vi "Set Minimum Pane Size to (0,0).vi"(8 "error in (no error)":errorcluster, 10 "Save VI (T)":bool=TRUE, 11 "vi path":path) -> (0 "error out":errorcluster)   [LabVIEW 2023]
uses:
  <vilib>/Utility/miscctls.llb/LVPointTypeDef.ctl
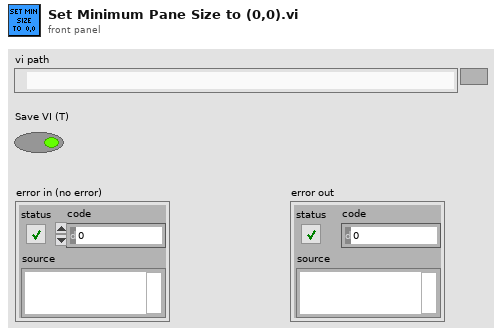
[diagram p1: front panel]
types:
  T1 = typedef "LVPointTypeDef.ctl" = cluster{"Horizontal":i16, "Vertical":i16}
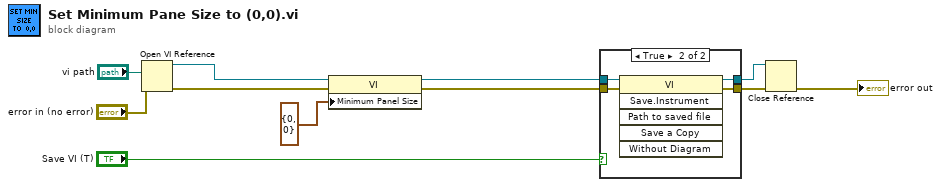
[diagram p0: block diagram]
diagram:
  n1 = Open VI Reference(vi path="vi path", error in (no error)="error in (no error)") -> (vi reference=w6:refnum<vi>, error out=w5:errorcluster)  [unwired: 4 in]
  n2 = property class="VI"(reference=w6, error in=w5, "Minimum Panel Size"=T1 {"Horizontal"=0, "Vertical"=0} ("Front Panel Window:Minimum Size")) -> (reference out=w4:refnum<vi>, error out=w2:errorcluster)
  n3 = case shown="True" "Save VI (T)" {
    tunnel: w2 -> [w13 w17]
    tunnel: [w13 w16] -> w9
    tunnel: [w12 w15] -> w8
    tunnel: w4 -> [w12 w14]
    frame False {
    }
    frame True {
      n4 = invoke class="VI" method="Save.Instrument"(reference=w14, error in=w17) -> (reference out=w15:refnum<vi>, error out=w16:errorcluster)  [unwired: 4 in, 4 out]
    }
  }
  n5 = Close Reference(reference=w8, error in (no error)=w9) -> (error out=→"error out":errorcluster)
